vi "mux1.vi"(0 "MUX S.n.":string, 2 "Ring":u16(ring) items=["Open All", "Ana Denge", "10R", "1R"], 3 "error in (no error)":errorcluster) -> (10 "error out":errorcluster)   [LabVIEW 2014]
uses:
  <vilib>/Utility/config.llb/Read Key (String).vi
  <vilib>/Utility/config.llb/NI_LVConfig.lvlib
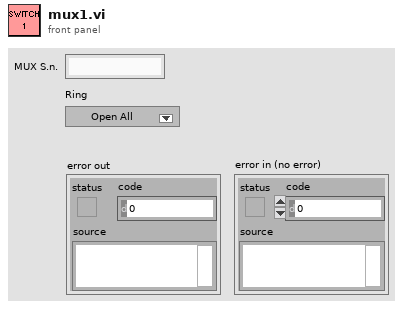
[diagram p1: front panel]
types:
  T1 = typedef "NI_LVConfig.lvlib/Config Data RefNum.ctl" = refnum<k1>
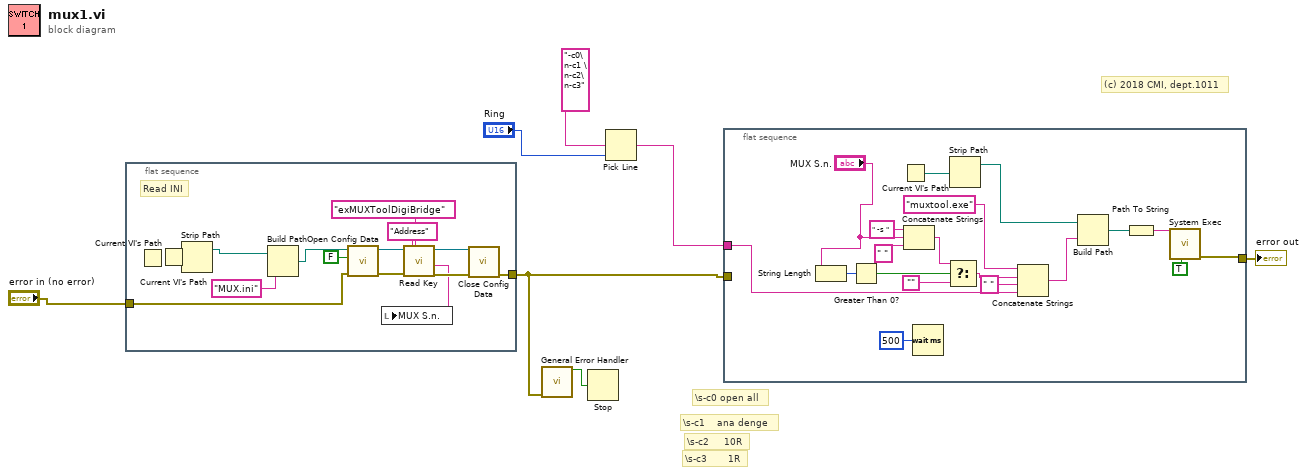
[diagram p0: block diagram]
diagram:
  # "\\s-c0 open all"
  # "\\s-c3       1R"
  # "\\s-c2     10R"
  # "\\s-c1    ana denge"
  # "(c) 2018 CMI, dept.1011"
  n1 = flat-sequence {
    tunnel: [w12] -> w3
    tunnel: "error in (no error)" -> [w8]
    frame #0 {
      # "Read INI"
      n2 = Current VI's Path() -> ()  [unwired: 1 out]
      n3 = Current VI's Path() -> (path=w10:path)
      n4 = Strip Path(path=w10) -> (stripped path=w9:path)  [unwired: 1 out]
      n5 = Build Path(base path=w9, name or relative path="MUX.ini") -> (appended path=w20:path)
      n6 = call <vilib>:"Open Config Data.vi"("error in (no error)"=w8, "create file if necessary (T)"=FALSE, "configuration file path"=w20) -> ("error out"=w18:errorcluster, "refnum"=w11:T1)  [unwired: 6 in, 1 out]
      n7 = call-poly <vilib>:"Read Key.vi"("section"="exMUXToolDigiBridge", "error in (no error)"=w18, "key"="Address", "refnum"=w11) -> ("error out"=w14:errorcluster, "value"=w13:string, "refnum out"=w15:T1)  [unwired: 4 in, 1 out]
      n8 = local write "MUX S.n."(w13) -> ()
      n9 = call <vilib>:"Close Config Data.vi"("error in (no error)"=w14, "refnum"=w15) -> ("error out"=w12:errorcluster)  [unwired: 8 in, 1 out]
    }
  }
  n10 = call <vilib>:"General Error Handler.vi"("error in (no error)"=w3) -> ("error?"=w5:bool)  [unwired: 10 in, 4 out]
  n11 = Stop(stop? (T)=w5) -> ()
  n12 = Pick Line(multi-line string="-c0\n-c1 \n-c2\n-c3", line index="Ring") -> (output string=w7:string)  [unwired: 1 in]
  n13 = flat-sequence {
    tunnel: w7 -> [w40]
    tunnel: w3 -> [_]
    tunnel: [w22] -> w2
    frame #0 {
      n14 = String Length(string="MUX S.n.") -> (length=w30:i32)
      n15 = Greater Than 0?(x=w30) -> (x > 0?=w29:bool)
      n16 = Current VI's Path() -> (path=w37:path)
      n17 = Concatenate Strings(" -s " ("string"), "MUX S.n.", " " ("string")) -> (w26:string)
      n18 = Wait (ms)(milliseconds to wait=u32 500) -> ()  [unwired: 1 out]
      n19 = Select(t=w26, s=w29, f="") -> (s? t:f=w31:string)
      n20 = Strip Path(path=w37) -> (stripped path=w36:path)  [unwired: 1 out]
      n21 = Concatenate Strings("muxtool.exe" ("name or relative path"), w31, " " ("string"), w40) -> (w33:string)
      n22 = Build Path(base path=w36, name or relative path=w33) -> (appended path=w39:path)
      n23 = Path To String(path=w39) -> (string=w38:string)
      n24 = call <vilib>:"System Exec.vi"("run minimized? (F)"=TRUE, "command line"=w38) -> ("error out"=w22:errorcluster)  [unwired: 6 in, 3 out]
    }
  }
  "error out" <- w2
